vi "Destroy Enqueuer.vi"(8 "error in (no error)":errorcluster, 11 "QDMH in":refnum<class "QDMH.lvclass">) -> (0 "error out":errorcluster, 3 "QDMH out":refnum<class "QDMH.lvclass">)   [LabVIEW 2023, in "QDMH.lvlib" / "QDMH.lvclass"]
doc: "This tool is designed to destroy localized queue references. \n\nThis does not completely eliminate the queue, elimination must be called by the master queue administrator, by calling force destroy queue."
uses:
  Library/QDMH.lvclass
  Library/QDMH.lvclass/QDMH.ctl
  Custom Controls/Message.ctl
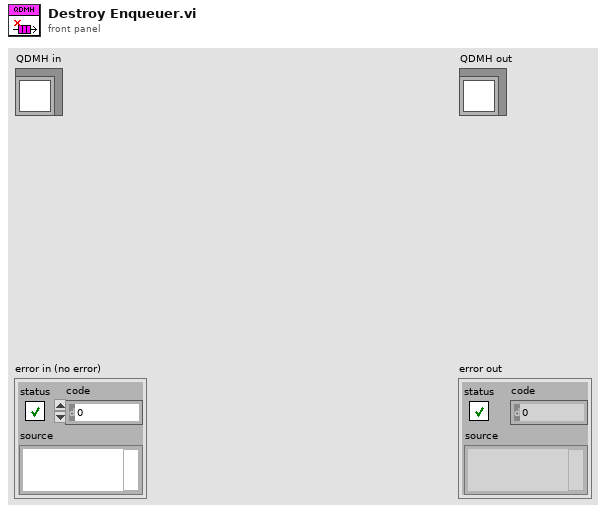
[diagram p1: front panel]
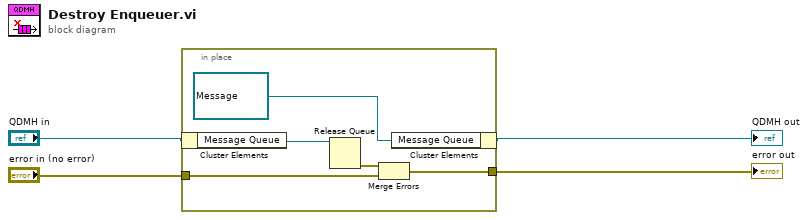
[diagram p0: block diagram]
diagram:
  n1 = in-place {
    in-place-border: "error in (no error)" -> [w6]
    in-place-border: [w5] -> w2
    n2 = in-place-cluster #1("QDMH in") -> ("Message Queue"=w9:refnum<queue>)
    n3 = Release Queue(queue=w9) -> (error out=w7:errorcluster)  [unwired: 2 in, 2 out]
    n4 = Merge Errors(w7, w6) -> (w5:errorcluster)
    n5 = in-place-cluster #1("Message Queue"=refnum<queue> refnum) -> (→"QDMH out":refnum<class "QDMH.lvclass">)
  }
  "error out" <- w2
